vi "Measurement_input_panel.vi"(0 "OK":T4, 2 "setup":T5, 5 "Setup filename":string) -> (11 "Setup filename out":string, 12 "Analysis Info cluster":T8[](array[typedef])=[{"Colour"=0, "Inst type"=enum."Pitot-static tube", "Inst name"="Manometer voltage", "Symbol"="U", "Code name"="", "Extra Info"="U", "Inst Array"=enum."PWA", "Extra Titles"=[], "Extra Values"=[], "U"=0.0, "u^2"=0.0, "u^3"=0.0, "u^4"=0.0, "Skew_u"=0.0, "Kurt_u"=0.0, "Sd Error in Mean"=0.0, "% u'/U"=0.0, "X"=0.0, "Y"=0.0, "Z"=0.0, "Timescale integral Estimate"=0.0, "Sd Error in Variance"=0.0, "Calib File"=path "", "Calib Constants"=[], "Output Position"=FALSE, "Full Stats"=FALSE, "Av Sampling Rate"=0.0, "Av No of Samples"=0.0, "Total Meas Time (s)"=0.0, "ADAM Ch Name"="", "Max value"=0.0, "Min value"=0.0, "Req Sample Rate Hz"=0.0, "Sync Delay Time (s)"=0.0, "Ch No"=0, "Device ID"="", "Use Latest Calib"=FALSE}, {"Colour"=0, "Inst type"=enum."Pitot-static tube", "Inst name"="Manometer voltage", "Symbol"="U", "Code name"="", "Extra Info"="U", "Inst Array"=enum."PWA", "Extra Titles"=[], "Extra Values"=[], "U"=0.0, "u^2"=0.0, "u^3"=0.0, "u^4"=0.0, "Skew_u"=0.0, "Kurt_u"=0.0, "Sd Error in Mean"=0.0, "% u'/U"=0.0, "X"=0.0, "Y"=0.0, "Z"=0.0, "Timescale integral Estimate"=0.0, "Sd Error in Variance"=0.0, "Calib File"=path "", "Calib Constants"=[], "Output Position"=FALSE, "Full Stats"=FALSE, "Av Sampling Rate"=0.0, "Av No of Samples"=0.0, "Total Meas Time (s)"=0.0, "ADAM Ch Name"="", "Max value"=0.0, "Min value"=0.0, "Req Sample Rate Hz"=0.0, "Sync Delay Time (s)"=0.0, "Ch No"=0, "Device ID"="", "Use Latest Calib"=FALSE}, {"Colour"=0, "Inst type"=enum."Pitot-static tube", "Inst name"="Manometer voltage", "Symbol"="U", "Code name"="", "Extra Info"="U", "Inst Array"=enum."PWA", "Extra Titles"=[], "Extra Values"=[], "U"=0.0, "u^2"=0.0, "u^3"=0.0, "u^4"=0.0, "Skew_u"=0.0, "Kurt_u"=0.0, "Sd Error in Mean"=0.0, "% u'/U"=0.0, "X"=0.0, "Y"=0.0, "Z"=0.0, "Timescale integral Estimate"=0.0, "Sd Error in Variance"=0.0, "Calib File"=path "", "Calib Constants"=[], "Output Position"=FALSE, "Full Stats"=FALSE, "Av Sampling Rate"=0.0, "Av No of Samples"=0.0, "Total Meas Time (s)"=0.0, "ADAM Ch Name"="", "Max value"=0.0, "Min value"=0.0, "Req Sample Rate Hz"=0.0, "Sync Delay Time (s)"=0.0, "Ch No"=0, "Device ID"="", "Use Latest Calib"=FALSE}] {"Sync Delay Time (s)" format="%.4f"; "Sd Error in Variance" format="%.2f"; "Skew_u" format="%.2f"; "% u'/U" format="%.2f"; "Sd Error in Mean" format="%.2f"; "Kurt_u" format="%.2f"; "u^4" format="%.2f"; "u^3" format="%.2f"; "U" format="%.2f"; "u^2" format="%.2f"})   [LabVIEW 2017]
uses:
  Controls/Inst_type.ctl
  Controls/Analysis_info_cluster.ctl
  Controls/Instrument_Array.ctl
  Controls/LDA_Setup.ctl
  Controls/Setup.ctl
  Controls/ok_button.ctl
  Controls/Trigger_Mode.ctl
  Controls/PWA_Data.ctl
  File/Setup_Filetype.ctl
  Controls/Post_Process.ctl
  Controls/App_Global.ctl
  Globals/Meas_global.vi
  Globals/Trav_pos_global.vi
  Globals/Preference_global.vi
  Globals/Dynamic_call_global.ph.vi
panel:
  in  "Edit temp and Press":bool
  in  "Acquisition Plug in":u16(ring) items=["7HP.vi", "ADAM_Server_Channels.vi", "DataTranslation.vi", "DT_With_Multiplexer.vi", "LDA_IP.vi", "Light_Power_Reading.vi", "LJ-T7DAQ.vi", "MAGIC_Pressures.vi", "Micro-Epsilon ILD1420.vi", "Na-DAS_7609.vi", "Na-DAS_and_MAGIC_Pressures.vi", "NI-DAQmx.vi", "NI-DAQmxBaseKernel.vi", "Pressure_Multiplexer.vi", "Simulate_kernal.vi"]
  in  "Select Duplicate Channels":bool
  in  "PWA Data":T1
  out "Inst type":T2
  out "Abs Press":dbl=1013.0 format="%.1fmBar"
  out "Temp":dbl=21.0 format="%.1fC"
  in  "Trigger mode":T3
  in  "Select Plug Ins":bool
  out "XW Present?":bool
  out "Read Setup File?":bool
  out "Setup Paths":string[](array[string])
  in  "Select ADAM Channels":bool
  in  "stop":bool
  out "Notes":string
  in  "Setup filename selector":u16(ring) items=["Current_Setup.xls", "LDA_UV_157.xls", "LDA_UW_157_Mirror.xls", "Micro-Epsilon_Height.xls", "Trav_Cam_Picture.xls", "Current_Setup.xls", "LDA_UW_157_Mirror.xls", "Micro-Epsilon_Height.xls", "Trav_Cam_Picture.xls"]
  in  "Synchronise Analogue channels with LDA":bool
  in  "LDA set up":T6={"dimensions"=enum."2D", "Sampling Rate Hz"=0.1}
  in  "LDA data":enum16{"No LDA data", "Take LDA data"}(ring)=enum."Take LDA data"
  in  "Cross wire":T7(ring)
  in  "No of Analogue inst":i32=1
  in  "Ch & spans choices":T10(array[cluster]) {"Sync Delay (ms)" min=0.0; "D" format="%.2f"; "Ch No" min=0}
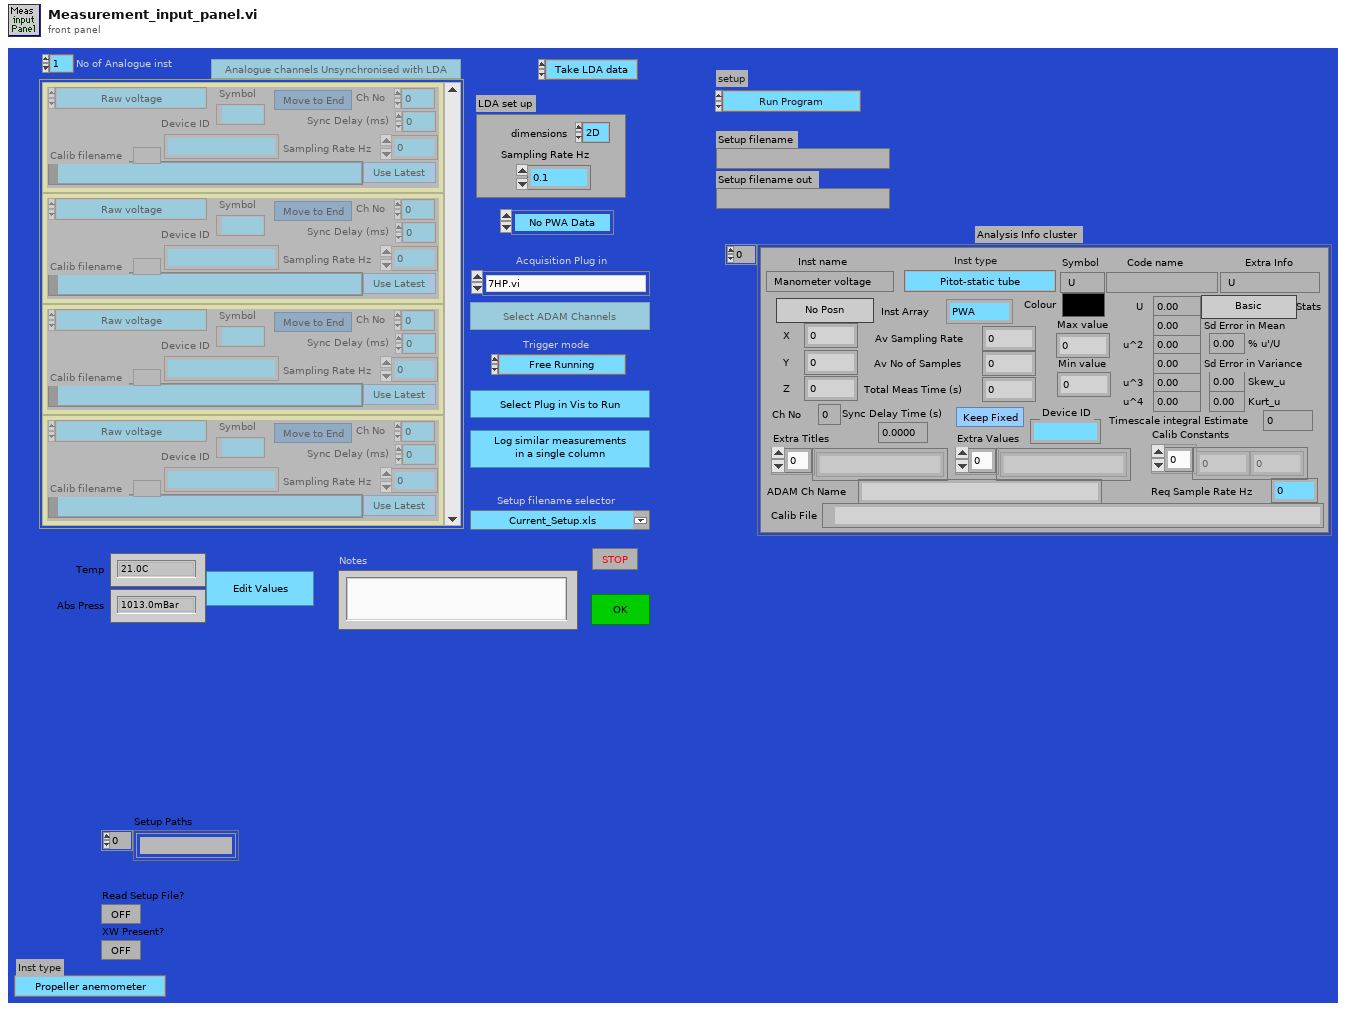
[diagram p1: front panel]
types:
  T1 = typedef "PWA_Data.ctl" = enum16{"No PWA Data", "One Ch PWA"}
  T2 = typedef "Inst_type.ctl" = enum16{"Propeller anemometer", "Raw voltage", "Pressure Transducer", "Pitot-static tube", "Preston tube", "Hot wire", "Cross wire 1", "Cross wire 2", "Generic Linear", "Generic Polynomial", "Generic BackPoly", "Fast FID", "Thermocouple", "Cold wire", "Pulsed Wire", "LDA Vel", "LDA Tran time", "LDA Arr time", "Microphone"}
  T3 = typedef "Trigger_Mode.ctl" = enum16{"Free Running", "Start on Trigger", "Trigger Every Block", "Trigger Every Sample"}
  T4 = typedef "ok_button.ctl" = bool
  T5 = typedef "Setup.ctl" = enum16{"Run Program", "Show Setup", "Save Current Setup", "Setup Front Panel"}
  T6 = typedef "LDA_Setup.ctl" = cluster{"dimensions":enum16{"1D", "2D"}, "Sampling Rate Hz":dbl}
  T7 = enum16{"2nd component as calculated", "2nd component multipled by -1"}
  T8 = typedef "Analysis_info_cluster.ctl" = cluster{"Colour":u32, "Inst type":T2, "Inst name":string, "Symbol":string, "Code name":string, "Extra Info":string, "Inst Array":T9, "Extra Titles":string[], "Extra Values":string[], "U":dbl, "u^2":dbl, "u^3":dbl, "u^4":dbl, "Skew_u":dbl, "Kurt_u":dbl, "Sd Error in Mean":dbl, "% u'/U":dbl, "X":dbl, "Y":dbl, "Z":dbl, "Timescale integral Estimate":dbl, "Sd Error in Variance":dbl, "Calib File":path, "Calib Constants":dbl[], "Output Position":bool, "Full Stats":bool, "Av Sampling Rate":dbl, "Av No of Samples":dbl, "Total Meas Time (s)":dbl, "ADAM Ch Name":string, "Max value":dbl, "Min value":dbl, "Req Sample Rate Hz":dbl, "Sync Delay Time (s)":dbl, "Ch No":i16, "Device ID":string, "Use Latest Calib":bool}
  T9 = typedef "Instrument_Array.ctl" = enum16{"PWA", "LDA", "Analogue"}
  T10 = cluster{"Ch No":i16, "Calib filename":path, "Inst type":T2, "Symbol":string, "Move channel":bool, "Use Latest":bool, "D":dbl, "Ch Name":string, "Sync Delay (ms)":dbl, "Device ID":string, "Sampling Rate Hz":dbl}[]
  T11 = typedef "Post_Process.ctl" = enum16{"Take New Data", "Post Process Raw Data File"}
  T12 = typedef "Setup_Filetype.ctl" = enum16{"Measurement Setups", "Calibration Setups", "General", "Results File Plotter Setups", "Speed Calib Tweaks"}
  T13 = typedef "App_Global.ctl" = enum16{"Read Global", "Write to Global", "Initialise Array"}
  T14 = enum16{"Zero or one", "One", "Zero or more", "One or more"}
  T15 = cluster{"Ch No":i16, "Calib filename":path, "Inst type":T2, "Symbol":string, "Move channel":bool, "Use Latest":bool, "D":dbl, "Ch Name":string, "Sync Delay (ms)":dbl, "Device ID":string, "Sampling Rate Hz":dbl}
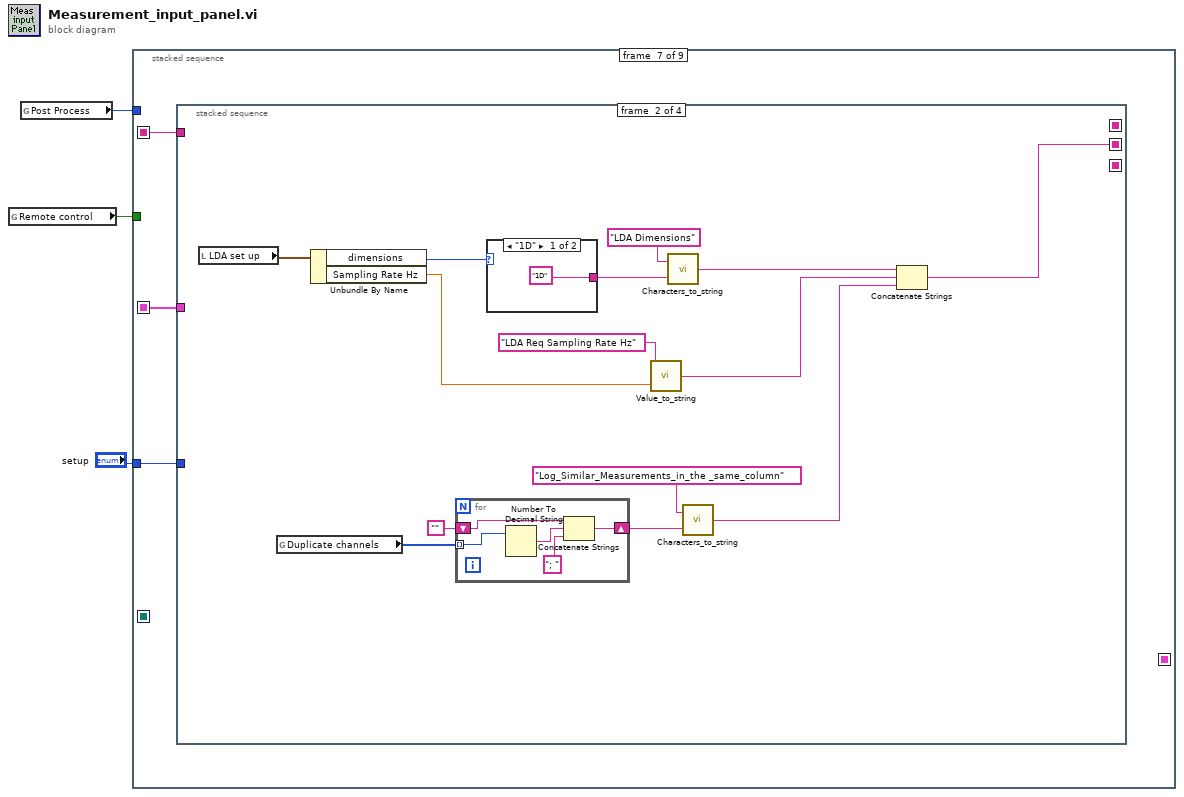
[diagram p0: block diagram]
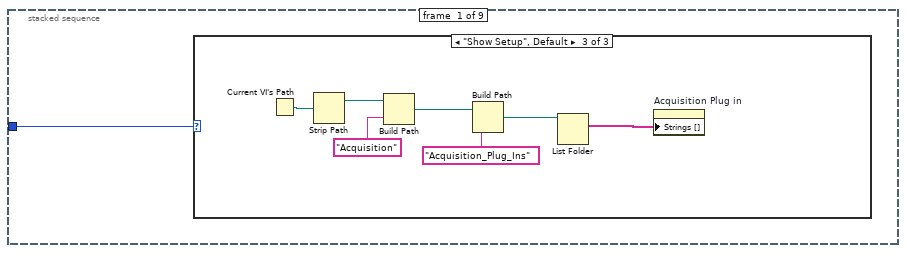
[diagram p2: hidden frame]
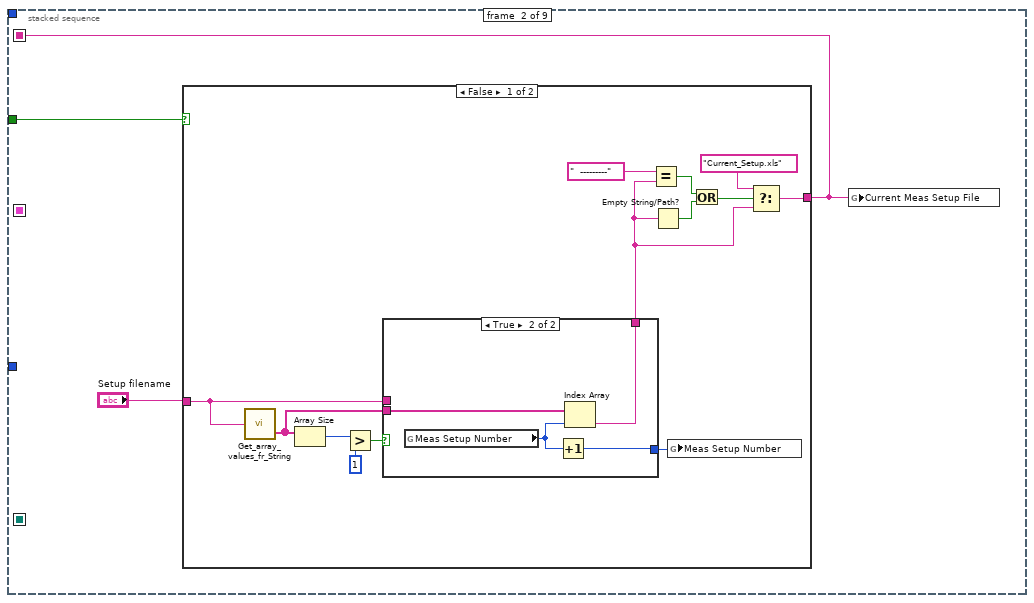
[diagram p5: hidden frame]
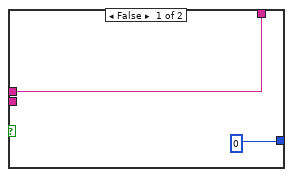
[diagram p6: hidden frame]
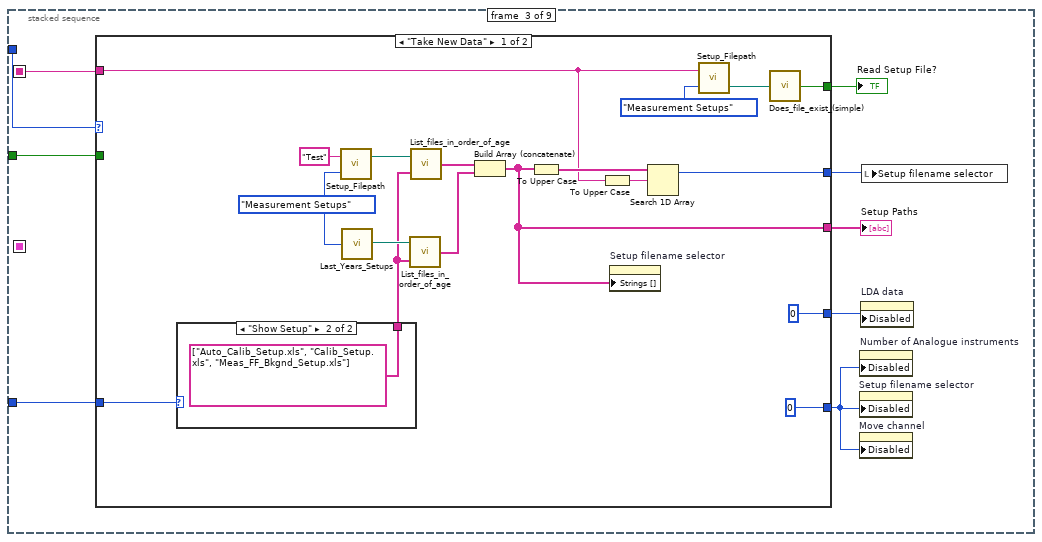
[diagram p8: hidden frame]
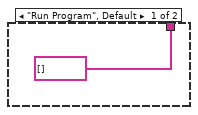
[diagram p9: hidden frame]
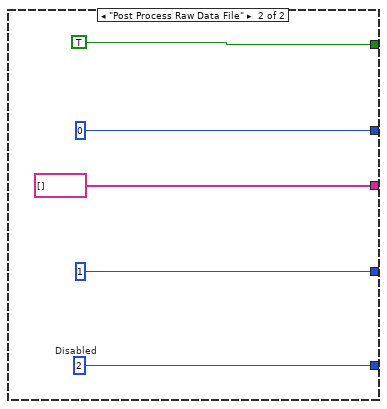
[diagram p10: hidden frame]
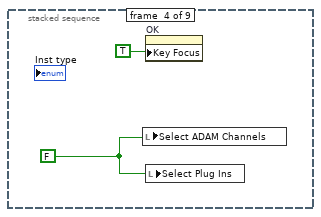
[diagram p11: hidden frame]
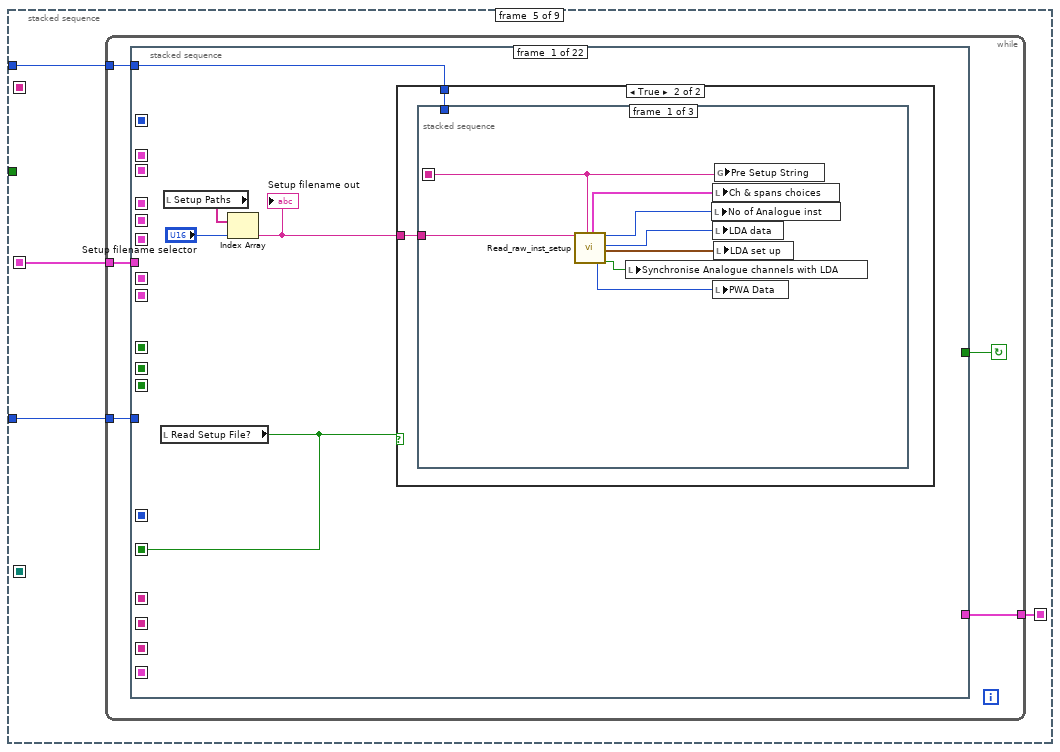
[diagram p12: hidden frame]
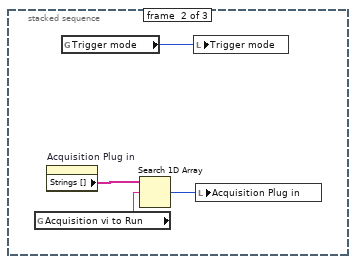
[diagram p14: hidden frame]
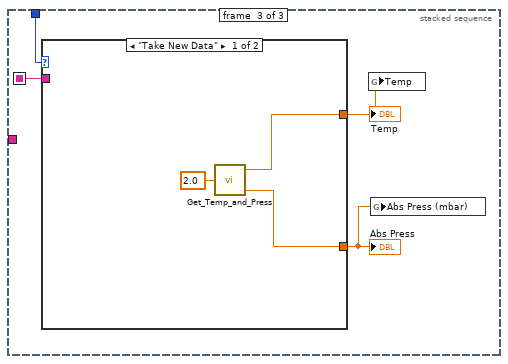
[diagram p15: hidden frame]
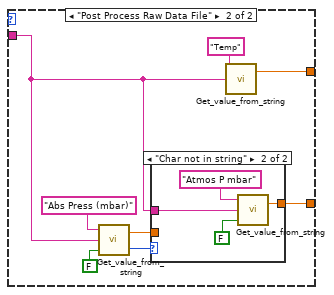
[diagram p16: hidden frame]
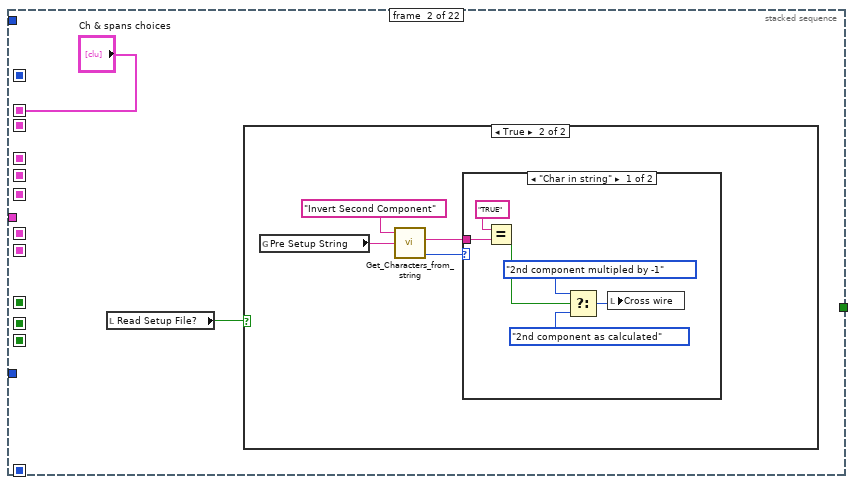
[diagram p18: hidden frame]
diagram:
  n1 = global read "Meas_global.vi" "Remote control"() -> (w1:bool)
  n2 = global read "Meas_global.vi" "Post Process"() -> (w3:T11)
  n3 = stacked-sequence {
    seq-local: [_ _ _ _ w74 _ _ _ _] -> [_ _ _ _ _ _ w699 w802 _]
    seq-local: [_ w13 _ _ _ _ _ _ _] -> [_ _ w35 _ _ _ w698 _ _]
    seq-local: [_ _ _ _ w71 _ _ _ _] -> [_ _ _ _ _ _ _ _ w855]
    seq-local: [_ _ _ _ _ _ _ w801 _] -> [_ _ _ _ _ _ _ _ w854]
    tunnel: w3 -> [_ _ w43 _ w73 _ _ w803 _]
    tunnel: "setup" -> [w4 _ w37 _ w72 _ w700 _ _]
    tunnel: w1 -> [_ w14 w36 _ _ _ _ _ _]
    frame #0 {
      n4 = case shown="\"Show Setup\", Default" w4 {
        frame "Run Program" {
        }
        frame "Setup Front Panel" {
        }
        frame "Show Setup", Default {
          n5 = Current VI's Path() -> (path=w11:path)
          n6 = Strip Path(path=w11) -> (stripped path=w10:path)  [unwired: 1 out]
          n7 = Build Path(base path=w10, name or relative path="Acquisition") -> (appended path=w7:path)
          n8 = Build Path(base path=w7, name or relative path="Acquisition_Plug_Ins") -> (appended path=w6:path)
          n9 = List Folder(path=w6) -> (filenames=w5:string[])  [unwired: 3 in, 3 out]
          n10 = property on="Acquisition Plug in" class="Ring (strict)"("Strings []"=w5) -> ()  [unwired: 2 in, 2 out]
        }
      }
    }
    frame #1 {
      n11 = case shown="False" w14 {
        tunnel: [w26 w34] -> w13
        tunnel: "Setup filename" -> [w15 w34]
        frame False {
          n12 = call "Get_array_values_fr_String.vi"("String Value"=w15) -> ("String array"=w17:string[])  [unwired: 1 out]
          n13 = Array Size(array=w17) -> (size(s)=w21:i32)
          n14 = Greater?(x=w21, y=1) -> (0:w19:bool)
          n15 = case shown="True" w19 {
            tunnel: [w29 w32] -> w18
            tunnel: w15 -> [w29 _]
            tunnel: w17 -> [_ w33]
            tunnel: [0 w30] -> w16
            frame False {
            }
            frame True {
              n16 = global read "Trav_pos_global.vi" "Meas Setup Number"() -> (w31:i32)
              n17 = Increment(x=w31) -> (x+1=w30:i32)
              n18 = Index Array(array=w33, index=w31) -> (element=w32:string)
            }
          }
          n19 = Equal?(x="  ---------" ("f"), y=w18) -> (x = y?=w25:bool)
          n20 = Empty String/Path?(string/path=w18) -> (empty?=w24:bool)
          n21 = global write "Trav_pos_global.vi" "Meas Setup Number"(w16) -> ()
          n22 = Or(x=w25, y=w24) -> (x .or. y?=w22:bool)
          n23 = Select(t="Current_Setup.xls", s=w22, f=w18) -> (s? t:f=w26:string)
        }
        frame True {
        }
      }
      n24 = global write "Trav_pos_global.vi" "Current Meas Setup File"(w13) -> ()
    }
    frame #2 {
      n25 = case shown="\"Take New Data\"" w43 {
        tunnel: [w44 string[] []] -> w39
        tunnel: [w57 TRUE ("exists")] -> w38
        tunnel: [u8 0 ("Disabled") w65] -> w40
        tunnel: [u8 0 ("Disabled") u8 1 ("Disabled")] -> w42
        tunnel: w35 -> [w53 _]
        tunnel: [w60 0 ("index of element")] -> w41
        tunnel: w37 -> [w55 _]
        tunnel: w36 -> [_ _]
        frame "Take New Data" {
          w47 = Setup_Filetype."Measurement Setups" ("Setup File Type")
          n26 = case shown="\"Show Setup\"" w55 {
            tunnel: [string[] [] ("file names") string[] ["Auto_Calib_Setup.xls", "Calib_Setup.xls", "Meas_FF_Bkgnd_Setup.xls"] ("file names")] -> w45
            frame "Run Program", Default {
            }
            frame "Show Setup" {
            }
          }
          n27 = call "Setup_Filepath.vi"("Setup File Type"=w47, "Filename in"="Test") -> ("Directory"=w48:path)  [unwired: 1 out]
          n28 = call "Last_Years_Setups.vi"("Setup File Type"=w47) -> ("Directory"=w46:path)
          n29 = call "List_files_in_order_of_age.vi"("Files to Hide"=w45, "Folder"=w46) -> ("file names"=w50:string[])
          n30 = call "List_files_in_order_of_age.vi"("Files to Hide"=w45, "Folder"=w48) -> ("file names"=w49:string[])
          n31 = Build Array (concatenate)(w49, w50) -> (w44:string[])
          n32 = To Upper Case(1:w44) -> (0:w59:string[])
          n33 = To Upper Case(1:w53) -> (0:w58:string)
          n34 = property on="Setup filename selector" class="Ring (strict)"("Strings []"=w44) -> ()  [unwired: 2 in, 2 out]
          n35 = Search 1D Array(1D array=w59, element=w58) -> (index of element=w60:i32)  [unwired: 1 out]
          n36 = call "Setup_Filepath.vi"("Setup File Type"=Setup_Filetype."Measurement Setups", "Filename in"=w53) -> ("Filename Out"=w52:path)  [unwired: 1 out]
          n37 = call "Does_file_exist_(simple).vi"("Pathname"=w52) -> ("exists?"=w57:bool)
        }
        frame "Post Process Raw Data File" {
          w65 = u8 2  # Disabled
        }
      }
      "Setup Paths" <- w39
      "Read Setup File?" <- w38
      n38 = property on="Number of Analogue instruments" class="DigNum (strict)"("Disabled"=w40) -> ()  [unwired: 2 in, 2 out]
      n39 = property on="Setup filename selector" class="Ring (strict)"("Disabled"=w40) -> ()  [unwired: 2 in, 2 out]
      n40 = property on="Move channel" class="Bool (strict)"("Disabled"=w40) -> ()  [unwired: 2 in, 2 out]
      n41 = property on="LDA data" class="Enum (strict)"("Disabled"=w42) -> ()  [unwired: 2 in, 2 out]
      n42 = local write "Setup filename selector"(w41) -> ()
    }
    frame #3 {
      w70 = FALSE ("Select Local ADAM Channels")
      n43 = local write "Select ADAM Channels"(w70) -> ()
      n44 = property on="OK" class="Bool"("Key Focus"=TRUE) -> ()  [unwired: 2 in, 2 out]
      n45 = local write "Select Plug Ins"(w70) -> ()
    }
    frame #4 {
      n46 = while {
        tunnel: w72 -> [w76]
        tunnel: w73 -> [w77]
        tunnel: [w79] -> w74
        tunnel: [w75] -> w71
        stop <- w78 continue-if-true
        n47 = stacked-sequence {
          seq-local: [_ _ _ _ _ _ _ _ w194 _ _ _ _ _ _ _ _ _ _ _ _ _] -> [_ _ _ _ _ _ _ _ _ _ w255 w280 w327 _ _ _ _ _ _ _ _ _]
          seq-local: [_ "Ch & spans choices" _ _ _ _ _ _ _ _ _ _ _ _ _ _ _ _ _ _ _ _] -> [_ _ _ _ _ w156 _ w190 w195 _ _ _ _ _ _ _ _ _ w556 _ _ _]
          seq-local: [_ _ _ _ _ w161 _ _ _ _ _ _ _ _ _ _ _ _ _ _ _ _] -> [_ _ _ _ _ _ _ _ w196 _ _ _ _ _ _ _ _ _ _ _ _ _]
          seq-local: [_ _ _ _ _ _ _ _ _ _ w257 _ _ _ _ _ _ _ _ _ _ _] -> [_ _ _ _ _ _ _ _ _ _ _ w281 _ _ _ _ _ _ _ _ _ w664]
          seq-local: [_ _ _ _ _ _ _ _ _ _ _ _ _ w359 _ _ _ _ _ _ _ _] -> [_ _ _ _ _ _ _ _ _ _ _ _ _ _ w378 _ _ _ _ _ _ _]
          seq-local: [_ _ _ _ _ _ _ _ _ _ _ _ _ _ w374 _ _ _ _ _ _ _] -> [_ _ _ _ _ _ _ _ _ _ _ _ _ _ _ w402 w472 _ _ _ w641 w665]
          seq-local: [_ _ _ _ _ _ _ _ _ _ _ w285 _ _ _ _ _ _ _ _ _ _] -> [_ _ _ _ _ _ _ _ _ _ _ _ _ w357 _ _ _ _ _ _ _ _]
          seq-local: [_ _ _ _ _ _ _ _ _ _ _ _ w331 _ _ _ _ _ _ _ _ _] -> [_ _ _ _ _ _ _ _ _ _ _ _ _ w356 _ _ _ _ _ _ _ _]
          seq-local: [_ _ _ _ _ _ _ _ _ w252 _ _ _ _ _ _ _ _ _ _ _ _] -> [_ _ _ _ _ _ _ _ _ _ w256 w282 _ _ _ _ _ _ _ _ _ w663]
          seq-local: [_ _ _ _ _ _ _ _ _ _ _ _ _ _ _ w401 _ _ _ _ _ _] -> [_ _ _ _ _ _ _ _ _ _ _ _ _ _ _ _ w475 _ _ _ _ _]
          seq-local: [_ _ _ _ _ _ _ _ _ _ _ _ _ _ _ w400 _ _ _ _ _ _] -> [_ _ _ _ _ _ _ _ _ _ _ _ _ _ _ _ w474 _ _ _ _ _]
          seq-local: [_ _ _ _ _ _ _ _ _ _ _ _ _ _ _ w399 _ _ _ _ _ _] -> [_ _ _ _ _ _ _ _ _ _ _ _ _ _ _ _ w473 _ _ _ _ _]
          seq-local: [_ _ _ _ _ _ _ _ _ _ _ _ _ _ _ _ w471 _ _ _ _ _] -> [_ _ _ _ _ _ _ _ _ _ _ _ _ _ _ _ _ _ _ w570 _ _]
          seq-local: [_ _ _ _ _ _ _ _ _ _ _ _ _ _ _ _ w469 _ _ _ _ _] -> [_ _ _ _ _ _ _ _ _ _ _ _ _ _ _ _ _ w516 _ _ _ _]
          seq-local: [w80 _ _ _ _ _ _ _ _ _ _ _ _ _ _ _ _ _ _ _ _ _] -> [_ _ _ _ _ _ _ _ _ _ _ _ _ _ _ _ w468 _ _ _ _ _]
          seq-local: [_ _ _ _ _ _ _ _ _ _ _ _ _ _ _ _ _ w515 _ _ _ _] -> [_ _ _ _ _ _ _ _ _ _ _ _ _ _ _ _ _ _ w557 _ _ _]
          seq-local: [_ _ _ _ _ _ _ _ _ _ _ _ _ _ _ _ _ _ w554 _ _ _] -> [_ _ _ _ _ _ _ _ _ _ _ _ _ _ _ _ _ _ _ w569 _ _]
          tunnel: [_ _ _ _ _ _ _ _ _ _ _ _ _ _ w374 _ _ _ _ _ _ _] -> w79
          tunnel: [_ _ _ _ _ _ _ _ _ _ _ w283 _ _ _ _ _ _ _ _ _ _] -> w78
          tunnel: w77 -> [w82 _ _ w135 _ _ _ _ _ w253 _ _ _ _ _ _ _ w526 _ _ _ _]
          tunnel: w76 -> [_ _ w131 _ w142 _ _ _ _ _ _ _ _ w358 _ _ _ _ _ w572 _ _]
          tunnel: [_ _ _ _ _ _ _ _ _ _ _ _ _ _ _ _ w471 _ _ _ _ _] -> w75
          frame #0 {
            n48 = local read "Read Setup File?"() -> (w80:bool)
            n49 = local read "Setup Paths"() -> (w84:string[])
            n50 = Index Array(array=w84, index="Setup filename selector") -> (element=w81:string)
            "Setup filename out" <- w81
            n51 = case shown="True" w80 {
              tunnel: w81 -> [_ w86]
              tunnel: w82 -> [_ w85]
              frame False {
              }
              frame True {
                n52 = stacked-sequence {
                  seq-local: [w89 _ _] -> [_ _ w101]
                  tunnel: w86 -> [w91 _ _]
                  tunnel: w85 -> [_ _ w102]
                  frame #0 {
                    n53 = call "Read_raw_inst_setup.vi"("Setup file"=w91) -> ("Setup string"=w89:string, "Ch & spans choices"=w87:T10, "PWA Data"=w88:T1, "Number of Analogue instruments"=w94:i32, "LDA data"=w93:enum16{"No LDA data", "Take LDA data"}, "LDA set up"=w90:T6, "Synchronise Analogue channels with LDA"=w92:bool)  [unwired: 12 out]
                    n54 = local write "Synchronise Analogue channels with LDA"(w92) -> ()
                    n55 = local write "No of Analogue inst"(w94) -> ()
                    n56 = local write "Ch & spans choices"(w87) -> ()
                    n57 = local write "LDA data"(w93) -> ()
                    n58 = local write "PWA Data"(w88) -> ()
                    n59 = local write "LDA set up"(w90) -> ()
                    n60 = global write "Meas_global.vi" "Pre Setup String"(w89) -> ()
                  }
                  frame #1 {
                    n61 = global read "Meas_global.vi" "Acquisition vi to Run"() -> (w96:string)
                    n62 = property on="Acquisition Plug in" class="Ring (strict)"() -> ("Strings []"=w97:string[])  [unwired: 2 in, 2 out]
                    n63 = global read "Meas_global.vi" "Trigger mode"() -> (w98:T3)
                    n64 = Search 1D Array(1D array=w97, element=w96) -> (index of element=w95:i32)  [unwired: 1 in]
                    n65 = local write "Trigger mode"(w98) -> ()
                    n66 = local write "Acquisition Plug in"(w95) -> ()
                  }
                  frame #2 {
                    n67 = case shown="\"Take New Data\"" w102 {
                      tunnel: w101 -> [_ w108]
                      tunnel: [w103 w107] -> w99
                      tunnel: [w104 w106] -> w100
                      frame "Take New Data" {
                        n68 = call "Get_Temp_and_Press.vi"("Averaging time (mins)"=2.0) -> ("Abs Press (mbar)"=w103:dbl, "Temperature"=w104:dbl)  [unwired: 3 out]
                      }
                      frame "Post Process Raw Data File" {
                        n69 = call "Get_value_from_string.vi"("Show Dialog?"=FALSE, "Input string"=w108, "Variable name"="Abs Press (mbar)") -> ("Status"=w112:enum16{"Char in string", "Char not in string"}, "Value"=w111:dbl)
                        n70 = case shown="\"Char not in string\"" w112 {
                          tunnel: [w114 w117] -> w107
                          tunnel: w111 -> [w114 _]
                          tunnel: w108 -> [_ w116]
                          frame "Char in string" {
                          }
                          frame "Char not in string" {
                            n71 = call "Get_value_from_string.vi"("Show Dialog?"=FALSE, "Input string"=w116, "Variable name"="Atmos P mbar") -> ("Value"=w117:dbl)  [unwired: 1 out]
                          }
                        }
                        n72 = call "Get_value_from_string.vi"("Input string"=w108, "Variable name"="Temp") -> ("Value"=w106:dbl)  [unwired: 1 in, 1 out]
                      }
                    }
                    "Abs Press" <- w99
                    "Temp" <- w100
                    n73 = global write "Meas_global.vi" "Temp"(w100) -> ()
                    n74 = global write "Meas_global.vi" "Abs Press (mbar)"(w99) -> ()
                  }
                }
              }
            }
          }
          frame #1 {
            n75 = local read "Read Setup File?"() -> (w120:bool)
            n76 = case shown="True" w120 {
              frame False {
              }
              frame True {
                n77 = global read "Meas_global.vi" "Pre Setup String"() -> (w123:string)
                n78 = call "Get_Characters_from_string.vi"("Input string"=w123, "Variable name"="Invert Second Component") -> ("Status"=w122:enum16{"Char in string", "Char not in string"}, "Value"=w121:string)  [unwired: 1 in]
                n79 = case shown="\"Char in string\"" w122 {
                  tunnel: w121 -> [w130 _]
                  frame "Char in string" {
                    n80 = Equal?(x="TRUE", y=w130) -> (x = y?=w126:bool)
                    n81 = Select(t=T7."2nd component multipled by -1" ("Cross wire/LDA"), s=w126, f=T7."2nd component as calculated" ("Cross wire/LDA")) -> (s? t:f=w128:T7)
                    n82 = local write "Cross wire"(w128) -> ()
                  }
                  frame "Char not in string" {
                  }
                }
              }
            }
          }
          frame #2 {
            n83 = case shown="\"Show Setup\"" w131 {
              frame "Run Program", Default {
              }
              frame "Show Setup" {
                n84 = property on="Acquisition Plug in" class="Ring (strict)"() -> ("Strings []"=w134:string[])  [unwired: 2 in, 2 out]
                n85 = Index Array(array=w134, index="Acquisition Plug in") -> (element=w132:string)
                n86 = global write "Meas_global.vi" "Acquisition vi to Run"(w132) -> ()
              }
            }
          }
          frame #3 {
            n87 = case shown="True" "Edit temp and Press" {
              tunnel: w135 -> [_ w137]
              frame False {
              }
              frame True {
                n88 = case shown="\"Take New Data\"" w137 {
                  frame "Take New Data" {
                    n89 = stacked-sequence {
                      frame #0 {
                        w138 = TRUE  # Wait until done
                        n90 = call "Run_Enter_Temp.vi"("Wait until done"=w138) -> ()  [unwired: 1 out]
                      }
                      frame #1 {
                        n91 = call "Get_Temp_and_Press.vi"("Averaging time (mins)"=2.0) -> ("Abs Press (mbar)"=w139:dbl, "Temperature"=w140:dbl)  [unwired: 3 out]
                        n92 = local write "Temp"(w140) -> ()
                        n93 = local write "Abs Press"(w139) -> ()
                      }
                    }
                  }
                  frame "Post Process Raw Data File" {
                  }
                }
              }
            }
          }
          frame #4 {
            n94 = case shown="True" "Select Plug Ins" {
              tunnel: w142 -> [_ w144]
              frame False {
              }
              frame True {
                n95 = stacked-sequence {
                  tunnel: w144 -> [w145 _]
                  frame #0 {
                    w149 = TRUE  # Show Panel?
                    n96 = global read "Meas_global.vi" "Pre Setup String"() -> (w148:string)
                    n97 = local write "Select Plug Ins"(FALSE ("Select Local ADAM Channels")) -> ()
                    n98 = call "Choose_Plug_In_to_Run.vi"("setup"=w145, "Show Panel?"=w149, "Setup String In"=w148) -> ("Setup String Out"=w147:string)  [unwired: 1 out]
                    n99 = global write "Meas_global.vi" "Pre Setup String"(w147) -> ()
                  }
                  frame #1 {
                    n100 = Current VI's Path() -> (path=w151:path)
                    n101 = call "Open_Close_Front_Panel.ph.vi"("Front Panel Window:Open"=TRUE, "VI path"=w151) -> ()  [unwired: 2 out]
                  }
                }
              }
            }
          }
          frame #5 {
            n102 = Initialize Array(0) -> (w163:i32[])  [unwired: 1 out]
            n103 = for {
              shift-right: [w170] -> w159
              shift-left: w163 -> [w171]
              tunnel: [w169] -> w157 mode=indexing
              tunnel: w156 -> [w168] mode=indexing
              tunnel: [w166] -> w155 mode=indexing
              n104 = Unbundle By Name(w168) -> ("Inst type"=w165:T2)
              n105 = case shown="\"LDA Vel\"" w165 {
                tunnel: w171 -> [w175 w179 w181 w185]
                tunnel: [w174 w178 w181 w184] -> w170
                tunnel: [FALSE TRUE FALSE FALSE] -> w169
                frame "Propeller anemometer", Default {
                  n106 = Build Array (concatenate)(w175, 1) -> (w174:i32[])
                }
                frame "Cross wire 1" {
                  n107 = Build Array (concatenate)(w179, 2) -> (w178:i32[])
                }
                frame "Cross wire 2" {
                }
                frame "LDA Vel" {
                  n108 = Build Array (concatenate)(w185, 1) -> (w184:i32[])
                }
              }
              n109 = Equal?(x=w165, y=Inst_type."Preston tube" ("Inst type")) -> (x = y?=w166:bool)
            }
            n110 = Or Array Elements(Boolean array=w155) -> (logical OR=w153:bool)
            n111 = Or Array Elements(Boolean array=w157) -> (logical OR=→"XW Present?":bool)
            n112 = property on="D" class="DigNum (strict)"("Visible"=w153) -> ()  [unwired: 2 in, 2 out]
            n113 = Build Array (concatenate)(w159, 1) -> (w158:i32[])
            n114 = Array Subset(array=w158, length="No of Analogue inst") -> (w162:i32[])  [unwired: 1 in]
            n115 = Add Array Elements(numeric array=w162) -> (sum=w161:i32)
          }
          frame #6 {
            "Notes" <- ""
          }
          frame #7 {
            n116 = Array Size(array=w190) -> (size(s)=w189:i32)
            n117 = Not Equal To 0?(x=w189) -> (x != 0?=w188:bool)
            n118 = case shown="True" w188 {
              tunnel: [enum16{"No Analogue data", "Take Analogue data"}."No Analogue data" ("Analogue data") enum16{"No Analogue data", "Take Analogue data"}."Take Analogue data" ("Analogue data")] -> w187
              frame False {
              }
              frame True {
              }
            }
            n119 = global write "Meas_global.vi" "Analogue data"(w187) -> ()
          }
          frame #8 {
            n120 = Index Array(array=w195, index=0) -> (element=w200:T15)
            n121 = Build Array (concatenate)(w195, w200) -> (w199:T10)
            n122 = Initialize Array(w200) -> (w198:T10)  [unwired: 1 out]
            n123 = for {
              N: w196 -> [_]
              tunnel: w199 -> [w208] mode=indexing
              shift-right: [w209] -> w194
              shift-left: w198 -> [w203]
              tunnel: Inst_type."Cross wire 2" ("Inst type") -> [w201]
              shift-right: [w207] -> _
              shift-left: _ -> [w206]
              tunnel: w199 -> [w205]
              n124 = Unbundle By Name(w208) -> ("Inst type"=w207:T2)
              n125 = Array Size(array=w203) -> (size(s)=w202:i32)
              n126 = Increment(x=w202) -> (x+1=w204:i32)
              n127 = case shown="\"Cross wire 1\"" w207 {
                tunnel: [w217 w237 w249] -> w209
                tunnel: w203 -> [w218 w239 w251]
                tunnel: w208 -> [w214 w240 w250]
                tunnel: w201 -> [w216 w244 _]
                tunnel: w206 -> [_ w243 _]
                tunnel: w205 -> [w221 _ _]
                tunnel: w204 -> [w220 _ _]
                frame "Cross wire 1" {
                  n128 = Index Array(array=w221, index=w220) -> (element=w215:T15)
                  n129 = Unbundle By Name(w215) -> ("Inst type"=w219:T2, "Sync Delay (ms)"=w212:dbl, "Ch No"=w211:i16, "Symbol"=w210:string)
                  n130 = Unbundle By Name(w214) -> ("Calib filename"=w213:path)
                  n131 = case shown="\"Cross wire 2\"" w219 {
                    tunnel: w218 -> [w230 w236]
                    tunnel: [w229 w235] -> w217
                    tunnel: w216 -> [w223 w231]
                    tunnel: w213 -> [w228 w234]
                    tunnel: w214 -> [w226 w232]
                    tunnel: w212 -> [w225 _]
                    tunnel: w211 -> [w224 _]
                    tunnel: w210 -> [w222 _]
                    frame "Cross wire 2" {
                      n132 = Bundle By Name(cluster=w226, "Calib filename"=w228, "Inst type"=w223, "Sync Delay (ms)"=w225, "Ch No"=w224, "Symbol"=w222) -> (w227:T15)
                      n133 = Build Array (concatenate)(w230, w226, w227) -> (w229:T10)
                    }
                    frame "Generic Linear", Default {
                      n134 = Bundle By Name(cluster=w232, "Calib filename"=w234, "Inst type"=w231) -> (w233:T15)
                      n135 = Build Array (concatenate)(w236, w232, w233) -> (w235:T10)
                    }
                  }
                }
                frame "Cross wire 2" {
                  n136 = Decrement(x=w244) -> (x-1=w242:T2)
                  n137 = Equal?(x=w242, y=w243) -> (x = y?=w241:bool)
                  n138 = Bundle By Name(cluster=w240, "Inst type"=w242) -> (w238:T15)
                  n139 = case shown="False" w241 {
                    tunnel: w239 -> [w247 w248]
                    tunnel: w238 -> [w246 _]
                    tunnel: [w245 w248] -> w237
                    frame False {
                      n140 = Build Array (concatenate)(w247, w246) -> (w245:T10)
                    }
                    frame True {
                    }
                  }
                }
                frame "Generic Linear", Default {
                  n141 = Build Array (concatenate)(w251, w250) -> (w249:T10)
                }
              }
            }
          }
          frame #9 {
            n142 = Equal?(x=w253, y=Post_Process."Take New Data" ("Post Process")) -> (x = y?=w252:bool)
          }
          frame #10 {
            n143 = case shown="True" "OK" {
              tunnel: w255 -> [_ w269]
              tunnel: [FALSE w260] -> w257
              tunnel: w256 -> [_ w261]
              frame False {
              }
              frame True {
                n144 = for {
                  tunnel: w269 -> [w279] mode=indexing
                  tunnel: [w275] -> w268 mode=indexing
                  n145 = Unbundle By Name(w279) -> ("Inst type"=w278:T2, "Symbol"=w277:string)
                  n146 = Number To Decimal String(number=w278) -> (decimal integer string=w276:string)  [unwired: 1 out]
                  n147 = Concatenate Strings(w276, w277) -> (w275:string)
                }
                n148 = call "Analyse_string_array.vi"("String array"=w268) -> ("Frequency"=w267:i32[])  [unwired: 2 out]
                n149 = Greater?(x=w267, y=1) -> (0:w265:bool[])
                n150 = global read "Meas_global.vi" "Remote control"() -> (w262:bool)
                n151 = Or Array Elements(Boolean array=w265) -> (logical OR=w264:bool)
                n152 = Compound Arithmetic op=AND(invert w262, w264, w261) -> (w263:bool)
                n153 = case shown="False" w263 {
                  tunnel: [TRUE FALSE] -> w260
                  frame False {
                  }
                  frame True {
                    n154 = Current VI's Path() -> (path=w272:path)
                    n155 = call "Open_Close_Front_Panel.ph.vi"("Front Panel Window:Open"=TRUE, "VI path"=w272) -> ()  [unwired: 2 out]
                    n156 = One Button Dialog(message="Non Unique symbol names") -> ()  [unwired: 2 out]
                  }
                }
              }
            }
          }
          frame #11 {
            n157 = And(x=w282, y=w281) -> (x .and. y?=w284:bool)
            n158 = case shown="True" w284 {
              tunnel: w280 -> [_ w293]
              tunnel: [FALSE w292] -> w285
              tunnel: [w286 w291] -> w283
              tunnel: w281 -> [w287 _]
              frame False {
                n159 = Not(x=w287) -> (.not. x?=w286:bool)
              }
              frame True {
                n160 = for {
                  shift-right: [w314] -> _
                  shift-left: string[] [] -> [w313]
                  tunnel: w293 -> [w311] mode=indexing
                  tunnel: [w302] -> w294 mode=indexing
                  shift-right: [w310] -> _
                  shift-left: path[] [] -> [w309]
                  n161 = Unbundle By Name(w311) -> ("Device ID"=w297:string, "Ch No"=w298:i16)
                  n162 = Unbundle By Name(w311) -> ("Inst type"=w308:T2, "Calib filename"=w305:path)
                  n163 = Format Into String(format string=" Ch %d", initial string=w297, w298) -> (resulting string=w295:string)  [unwired: 1 in, 1 out]
                  n164 = Equal?(x=Inst_type."Fast FID" ("Inst type"), y=w308) -> (x = y?=w301:bool)
                  n165 = Search 1D Array(1D array=w313, element=w295) -> (index of element=w312:i32)  [unwired: 1 out]
                  n166 = Search 1D Array(1D array=w309, element=w305) -> (index of element=w306:i32)  [unwired: 1 out]
                  n167 = Greater Or Equal To 0?(x=w306) -> (x >= 0?=w300:bool)
                  n168 = case shown="0, Default" w312 {
                    tunnel: w295 -> [w325 _]
                    tunnel: [w321 FALSE ("true")] -> w304
                    frame 0, Default {
                      n169 = Format Into String(format string="The Channel %s appears more than once", w325) -> (resulting string=w323:string)  [unwired: 2 in, 1 out]
                      n170 = One Button Dialog(message=w323, button name ("OK")="Ok") -> (true=w321:bool)
                    }
                    frame -1 {
                    }
                  }
                  n171 = And(x=w300, y=w301) -> (x .and. y?=w299:bool)
                  n172 = case shown="True" w299 {
                    tunnel: [w316 FALSE ("true")] -> w303
                    tunnel: w305 -> [w315 _]
                    frame True {
                      n173 = Format Into String(format string="Calibration file %s is used more than once.", w315) -> (resulting string=w318:string)  [unwired: 2 in, 1 out]
                      n174 = One Button Dialog(message=w318, button name ("OK")="Ok") -> (true=w316:bool)
                    }
                    frame False {
                    }
                  }
                  n175 = Build Array (concatenate)(w313, w295) -> (w314:string[])
                  n176 = Build Array (concatenate)(w309, w305) -> (w310:path[])
                  n177 = Or(x=w304, y=w303) -> (x .or. y?=w302:bool)
                }
                n178 = Or Array Elements(Boolean array=w294) -> (logical OR=w291:bool)
                n179 = Not(x=w291) -> (.not. x?=w292:bool)
              }
            }
          }
          frame #12 {
            n180 = call "Current_Calib_Filenames.vi"("Mode"=App_Global."Read Global") -> ("Calib Filename Out"=w328:path[], "Channel Numbers Out"=w329:i16[])  [unwired: 2 in, 1 out]
            n181 = for {
              tunnel: w327 -> [w342] mode=indexing
              tunnel: w329 -> [w344]
              tunnel: w328 -> [w343]
              tunnel: [w341] -> w331 mode=indexing
              n182 = Unbundle By Name(w342) -> ("Inst type"=w334:T2, "Ch No"=w336:i16, "Use Latest"=w337:bool, "Inst type"=w340:T2)
              n183 = Not Equal?(x=w340, y=Inst_type."Cross wire 2" ("Inst type")) -> (x != y?=w338:bool)
              n184 = Not Equal?(x=Inst_type."Raw voltage" ("Inst type"), y=w334) -> (x != y?=w332:bool)
              n185 = Compound Arithmetic op=AND(w337, w338) -> (w335:bool)
              n186 = case shown="True" w335 {
                tunnel: w344 -> [_ w355]
                tunnel: w336 -> [_ w354]
                tunnel: w343 -> [_ w352]
                tunnel: w342 -> [w345 w351]
                tunnel: [w345 w350] -> w341
                tunnel: w332 -> [_ w347]
                frame False {
                }
                frame True {
                  n187 = Search 1D Array(1D array=w355, element=w354) -> (index of element=w353:i32)  [unwired: 1 out]
                  n188 = Index Array(array=w352, index=w353) -> (element=w348:path)
                  n189 = Select(t=w348, s=w347, f=path "") -> (s? t:f=w349:path)
                  n190 = Bundle By Name(cluster=w351, "Calib filename"=w349) -> (w350:T15)
                }
              }
            }
          }
          frame #13 {
            n191 = case shown="True" w357 {
              tunnel: w356 -> [w360 w363]
              tunnel: [w360 w362] -> w359
              tunnel: w358 -> [_ w361]
              frame False {
              }
              frame True {
                n192 = case shown="\"Run Program\", Default" w361 {
                  tunnel: w363 -> [w365 w373]
                  tunnel: [w364 w373] -> w362
                  frame "Run Program", Default {
                    n193 = for {
                      tunnel: w365 -> [w366] mode=indexing
                      tunnel: [w367] -> w364 mode=indexing
                      n194 = Unbundle By Name(w366) -> ("Calib filename"=w372:path, "Use Latest"=w371:bool, "Ch No"=w370:i16, "Inst type"=w369:T2)
                      n195 = call "Find_calibration_file.vi"("Inst type"=w369, "Ch No"=w370, "Use Latest Calib"=w371, "filename"=w372) -> ("filename out"=w368:path)
                      n196 = Bundle By Name(cluster=w366, "Calib filename"=w368) -> (w367:T15)
                    }
                  }
                  frame "Setup Front Panel" {
                  }
                }
              }
            }
          }
          frame #14 {
            w376 = 0 ("Index")
            n197 = Index Array(array=w378, index=w376) -> (element=w377:T15)
            n198 = Initialize Array(w377, w376) -> (w375:T10)
            n199 = for {
              shift-right: [w386] -> w380
              shift-left: w375 -> [w385]
              shift-right: [w387] -> w381
              shift-left: w375 -> [w389]
              tunnel: w378 -> [w388] mode=indexing
              n200 = Unbundle By Name(w388) -> ("Move channel"=w390:bool)
              n201 = case shown="False" w390 {
                tunnel: w389 -> [w392 w398]
                tunnel: w388 -> [w394 w397]
                tunnel: [w393 w398] -> w387
                tunnel: [w391 w396] -> w386
                tunnel: w385 -> [w391 w395]
                frame False {
                  n202 = Build Array (concatenate)(w392, w394) -> (w393:T10)
                }
                frame True {
                  n203 = Build Array (concatenate)(w395, w397) -> (w396:T10)
                }
              }
            }
            n204 = Build Array (concatenate)(w381, w380) -> (w379:T10)
            n205 = for {
              tunnel: w379 -> [w384] mode=indexing
              tunnel: [w382] -> w374 mode=indexing
              n206 = Bundle By Name(cluster=w384, "Move channel"=FALSE) -> (w382:T15)
            }
          }
          frame #15 {
            # "#ToDo Maybe make this more generic..?"
            n207 = for {
              shift-right: [w408] -> _
              shift-left: string[] [] -> [w409]
              tunnel: [w411] -> w400 mode=indexing
              tunnel: [w405] -> w401 mode=indexing
              tunnel: w402 -> [w407] mode=indexing
              tunnel: [w404] -> w399 mode=indexing
              n208 = Unbundle By Name(w407) -> ("Inst type"=w410:T2)
              n209 = case shown="\"Raw voltage\"" w410 {
                tunnel: [w418 w422 w425 w429 w433 w437 w441 "XW" w448 w452 w457 w460 w464] -> w405
                tunnel: ["U" "P" "U" "U" "tau" "U" "U" "W" "U" "V" "C" "T" "T"] -> w412
                tunnel: w409 -> [w419 w423 w427 w431 w435 w439 w443 w445 w450 w454 w458 w462 w466]
                tunnel: [w417 w421 w426 w430 w434 w438 w442 w445 w449 w453 w456 w461 w465] -> w408
                frame "Propeller anemometer" {
                  w418 = "Prop"
                  n210 = Build Array (concatenate)(w419, w418) -> (w417:string[])
                }
                frame "Pressure Transducer" {
                  w422 = "Mano"
                  n211 = Build Array (concatenate)(w423, w422) -> (w421:string[])
                }
                frame "Raw voltage" {
                  w425 = "RV"
                  n212 = Build Array (concatenate)(w427, w425) -> (w426:string[])
                }
                frame "Pitot-static tube" {
                  w429 = "Pitot"
                  n213 = Build Array (concatenate)(w431, w429) -> (w430:string[])
                }
                frame "Preston tube" {
                  w433 = "Preston"
                  n214 = Build Array (concatenate)(w435, w433) -> (w434:string[])
                }
                frame "Hot wire" {
                  w437 = "HW"
                  n215 = Build Array (concatenate)(w439, w437) -> (w438:string[])
                }
                frame "Cross wire 1" {
                  w441 = "XW"
                  n216 = Build Array (concatenate)(w443, w441) -> (w442:string[])
                }
                frame "Cross wire 2" {
                }
                frame "Generic Linear", Default {
                  w448 = "Gen"
                  n217 = Build Array (concatenate)(w450, w448) -> (w449:string[])
                }
                frame "Microphone" {
                  w452 = "Mic"
                  n218 = Build Array (concatenate)(w454, w452) -> (w453:string[])
                }
                frame "Fast FID" {
                  w457 = "FF"
                  n219 = Build Array (concatenate)(w458, w457) -> (w456:string[])
                }
                frame "Thermocouple" {
                  w460 = "T"
                  n220 = Build Array (concatenate)(w462, w460) -> (w461:string[])
                }
                frame "Cold wire" {
                  w464 = "CW"
                  n221 = Build Array (concatenate)(w466, w464) -> (w465:string[])
                }
              }
              n222 = call "Analyse_string_array.vi"("String array"=w408) -> ("Unique strings"=w416:string[], "Frequency"=w414:i32[])  [unwired: 1 out]
              n223 = Search 1D Array(1D array=w416, element=w405) -> (index of element=w415:i32)  [unwired: 1 out]
              n224 = Index Array(array=w414, index=w415) -> (element=w406:i32)
              n225 = Number To Decimal String(number=w406) -> (decimal integer string=w404:string)  [unwired: 1 out]
              n226 = Concatenate Strings(w404, w405, ":", w412) -> (w411:string)
            }
          }
          frame #16 {
            w476 = T8 {"Colour"=0, "Inst type"=enum."Pitot-static tube", "Inst name"="Manometer voltage", "Symbol"="U", "Code name"="", "Extra Info"="U", "Inst Array"=enum."PWA", "Extra Titles"=[], "Extra Values"=[], "U"=0.0, "u^2"=0.0, "u^3"=0.0, "u^4"=0.0, "Skew_u"=0.0, "Kurt_u"=0.0, "Sd Error in Mean"=0.0, "% u'/U"=0.0, "X"=0.0, "Y"=0.0, "Z"=0.0, "Timescale integral Estimate"=0.0, "Sd Error in Variance"=0.0, "Calib File"=path "", "Calib Constants"=[], "Output Position"=FALSE, "Full Stats"=FALSE, "Av Sampling Rate"=0.0, "Av No of Samples"=0.0, "Total Meas Time (s)"=0.0, "ADAM Ch Name"="", "Max value"=0.0, "Min value"=0.0, "Req Sample Rate Hz"=0.0, "Sync Delay Time (s)"=0.0, "Ch No"=0, "Device ID"="", "Use Latest Calib"=FALSE}  # Analysis info cluster
            n227 = global read "Meas_global.vi" "Pre Setup String"() -> (w470:string)
            n228 = for {
              tunnel: w472 -> [w490] mode=indexing
              tunnel: w475 -> [w504] mode=indexing
              tunnel: [w506] -> w471 mode=indexing
              tunnel: w474 -> [w493] mode=indexing
              tunnel: w476 -> [w505]
              tunnel: w473 -> [w501] mode=indexing
              tunnel: w470 -> [w494]
              tunnel: [w489] -> w469 mode=indexing
              tunnel: w468 -> [w485]
              n229 = Unbundle By Name(w490) -> ("Use Latest"=w477:bool, "Sync Delay (ms)"=w483:dbl, "Ch No"=w478:i16, "Inst type"=w499:T2, "Symbol"=w498:string, "D"=w497:dbl, "Ch Name"=w486:string, "Device ID"=w480:string, "Sampling Rate Hz"=w479:dbl)
              n230 = Empty String/Path?(string/path=w498) -> (empty?=w502:bool)
              n231 = Concatenate Strings(w493, "_ADAM_Ch_Name" ("string")) -> (w491:string)
              n232 = Select(t=w501, s=w502, f=w498) -> (s? t:f=w500:string)
              n233 = Format Into String(format string="%s (%s)" ("Format String"), w504, w500) -> (resulting string=w495:string)  [unwired: 2 in, 1 out]
              n234 = call "Get_Characters_from_string.vi"("Input string"=w494, "Variable name"=w491) -> ("Value"=w488:string)  [unwired: 1 in, 1 out]
              n235 = Select(t=w488, s=w485, f=w486) -> (s? t:f=w487:string)
              n236 = Bundle By Name(cluster=w490, "Ch Name"=w487) -> (w489:T15)
              n237 = case shown="\"Preston tube\"" w499 {
                tunnel: [w509 w512] -> w481
                tunnel: w478 -> [w507 _]
                tunnel: w497 -> [_ w510]
                frame "Propeller anemometer", Default {
                  n238 = Format Into String(format string="Ch %d" ("Format String"), w507) -> (resulting string=w509:string)  [unwired: 2 in, 1 out]
                }
                frame "Preston tube" {
                  n239 = Format Into String(format string="D = %.2f" ("Format String"), w510) -> (resulting string=w512:string)  [unwired: 2 in, 1 out]
                }
              }
              n240 = Divide(x=w483, y=1000.0) -> (x/y=w482:dbl)
              n241 = Bundle By Name(cluster=w505, "Use Latest Calib"=w477, "Extra Info"=w481, "Device ID"=w480, "Inst type"=w499, "Inst name"=w495, "Symbol"=w500, "Code name"=w493, "Inst Array"=Instrument_Array."Analogue", "ADAM Ch Name"=w487, "Sync Delay Time (s)"=w482, "Req Sample Rate Hz"=w479, "Ch No"=w478) -> (w506:T8)
            }
          }
          frame #17 {
            w523 = u8 0  # Disabled
            n242 = global read "Meas_global.vi" "Acquisition vi to Run"() -> (w519:string)
            n243 = local read "Read Setup File?"() -> (w520:bool)
            n244 = Equal?(x="ADAM_Server_Channels.vi", y=w519) -> (x = y?=w517:bool)
            n245 = And(x=w520, y=w517) -> (x .and. y?=w529:bool)
            n246 = Or(x="Select ADAM Channels", y=w529) -> (x .or. y?=w524:bool)
            n247 = Equal?(x=w526, y=Post_Process."Take New Data" ("Post Process")) -> (x = y?=w525:bool)
            n248 = And(x=w525, y=w524) -> (x .and. y?=w514:bool)
            n249 = case shown="True" w514 {
              tunnel: [w530 w531] -> w515
              tunnel: w516 -> [w530 w534]
              tunnel: "Select ADAM Channels" -> [_ w533]
              tunnel: w517 -> [_ w532]
              frame False {
              }
              frame True {
                n250 = stacked-sequence {
                  seq-local: [w536 _ _] -> [_ w546 _]
                  tunnel: w534 -> [w538 w545 _]
                  tunnel: [_ w543 _] -> w531
                  tunnel: w533 -> [w540 _ w552]
                  tunnel: w532 -> [w539 _ _]
                  frame #0 {
                    n251 = Not(x=w539) -> (.not. x?=w535:bool)
                    n252 = Array Size(array=w538) -> ()  [unwired: 1 out]
                    n253 = for {
                      tunnel: w538 -> [w542] mode=indexing
                      tunnel: [w541] -> w537 mode=indexing
                      n254 = Unbundle By Name(w542) -> ("Ch Name"=w541:string)
                    }
                    n255 = call "Get_local_ADAM_Chs.vi"("Local ADAM?"=w535, "Show setup"=w540, "Desired ADAM Channels"=w537) -> ("Chosen Channels"=w536:string[])  [unwired: 1 out]
                  }
                  frame #1 {
                    n256 = for {
                      tunnel: [w551] -> w543 mode=indexing
                      tunnel: w546 -> [w550] mode=indexing
                      tunnel: w545 -> [w549]
                      i -> [w548]
                      n257 = Index Array(array=w549, index=w548) -> (element=w547:T15)
                      n258 = Bundle By Name(cluster=w547, "Ch No"=w548, "Ch Name"=w550) -> (w551:T15)
                    }
                    n259 = Array Size(array=w543) -> (size(s)=w544:i32)
                    n260 = local write "No of Analogue inst"(w544) -> ()
                  }
                  frame #2 {
                    n261 = case shown="True" w552 {
                      frame False {
                      }
                      frame True {
                        n262 = local write "Select ADAM Channels"(FALSE ("Select Local ADAM Channels")) -> ()
                      }
                    }
                  }
                }
              }
            }
            n263 = Not(x=w517) -> (.not. x?=w513:bool)
            n264 = Select(t=w523, s=w517, f=u8 2 ("Disabled")) -> (s? t:f=w521:u8)
            n265 = property on="Select ADAM Channels" class="Bool (strict)"("Disabled"=w521) -> ()  [unwired: 2 in, 2 out]
            n266 = property on="Ch Name" class="Str"("Visible"=w517) -> ()  [unwired: 2 in, 2 out]
            n267 = property on="Ch No" class="DigNum (strict)"("Visible"=w513) -> ()  [unwired: 2 in, 2 out]
            n268 = property on="Device ID" class="Str"("Visible"=w513) -> ()  [unwired: 2 in, 2 out]
            n269 = property on="Sampling Rate Hz" class="DigNum (strict)"("Visible"=w513) -> ()  [unwired: 2 in, 2 out]
          }
          frame #18 {
            n270 = Not Equal?(x=w556, y=w557) -> (x != y?=w558:bool)
            n271 = local read "LDA data"() -> (w555:enum16{"No LDA data", "Take LDA data"})
            n272 = case shown="True" w558 {
              tunnel: w557 -> [_ w565]
              frame False {
              }
              frame True {
                n273 = local write "Ch & spans choices"(w565) -> ()
              }
            }
            n274 = case shown="\"Take LDA data\"" w555 {
              tunnel: [0 w560] -> w554
              frame "No LDA data" {
              }
              frame "Take LDA data" {
                n275 = local read "LDA set up"() -> (w562:T6)
                n276 = Unbundle By Name(w562) -> ("dimensions"=w561:enum16{"1D", "2D"})
                n277 = case shown="\"2D\"" w561 {
                  tunnel: [1 2] -> w560
                  frame "1D" {
                  }
                  frame "2D" {
                  }
                }
              }
            }
          }
          frame #19 {
            n278 = global read "Meas_global.vi" "Duplicate channels"() -> (w568:i32[])
            n279 = case shown="False" "Select Duplicate Channels" {
              tunnel: w572 -> [_ _]
              tunnel: w570 -> [w583 w607]
              tunnel: w568 -> [w577 w609]
              tunnel: [w576 w608] -> w567
              tunnel: w569 -> [w575 w606]
              frame False {
                n280 = for {
                  tunnel: w583 -> [w603] mode=indexing
                  tunnel: [w602] -> w574 mode=indexing
                  n281 = Unbundle By Name(w603) -> ("Inst type"=w602:T2)
                }
                n282 = case shown="1" w575 {
                  tunnel: [w592 w594 w597] -> w573
                  tunnel: w574 -> [w592 w595 w598]
                  frame 0, Default {
                  }
                  frame 1 {
                    n283 = Build Array (concatenate)(Inst_type."LDA Vel" ("Inst type"), w595) -> (w594:T2[])
                  }
                  frame 2 {
                    w596 = Inst_type."LDA Vel" ("Inst type")
                    n284 = Build Array (concatenate)(w596, w596, w598) -> (w597:T2[])
                  }
                }
                n285 = for {
                  tunnel: w577 -> [w599] mode=indexing
                  tunnel: w573 -> [w601]
                  tunnel: [w600] -> w587 mode=indexing
                  tunnel: [w599] -> w584 mode=indexing
                  n286 = Index Array(array=w601, index=w599) -> (element=w600:T2)
                }
                n287 = Array Size(array=w573) -> (size(s)=w585:i32)
                n288 = Array Max & Min(array=w587) -> (max value=w588:T2, min value=w589:T2)  [unwired: 2 out]
                n289 = Array Max & Min(array=w584) -> (max index (indices)=w586:i32)  [unwired: 3 out]
                n290 = Array Size(array=w577) -> (size(s)=w582:i32)
                n291 = Greater?(x=w582, y=1) -> (0:w579:bool)
                n292 = Equal?(x=w588, y=w589) -> (x = y?=w591:bool)
                n293 = Greater?(x=w585, y=w586) -> (0:w590:bool)
                n294 = Compound Arithmetic op=AND(w579, w591, w590) -> (w578:bool)
                n295 = Select(t=w577, s=w578, f=i32[] [] ("32bit integer")) -> (s? t:f=w576:i32[])
              }
              frame True {
                n296 = for {
                  tunnel: w607 -> [w625] mode=indexing
                  tunnel: [w624] -> w604 mode=indexing
                  n297 = Unbundle By Name(w625) -> ("Inst name"=w624:string)
                }
                n298 = case shown="1" w606 {
                  tunnel: [w616 w618 w622] -> w605
                  tunnel: w604 -> [w616 w619 w623]
                  frame 0, Default {
                  }
                  frame 1 {
                    n299 = Build Array (concatenate)("1st LDA Ch", w619) -> (w618:string[])
                  }
                  frame 2 {
                    n300 = Build Array (concatenate)("1st LDA Ch", "2nd LDA Ch", w623) -> (w622:string[])
                  }
                }
                n301 = for {
                  shift-right: [w627] -> w612
                  shift-left: string[] [] -> [w628]
                  tunnel: w609 -> [w630]
                  tunnel: [w626] -> w611 mode=indexing
                  tunnel: w605 -> [w626] mode=indexing
                  i -> [w631]
                  n302 = Search 1D Array(1D array=w630, element=w631) -> (index of element=w629:i32)  [unwired: 1 out]
                  n303 = case shown="0, Default" w629 {
                    tunnel: w628 -> [w634 w635]
                    tunnel: w626 -> [w633 _]
                    tunnel: [w632 w635] -> w627
                    frame 0, Default {
                      n304 = Build Array (concatenate)(w634, w633) -> (w632:string[])
                    }
                    frame -1 {
                    }
                  }
                }
                n305 = local write "Select Duplicate Channels"(FALSE ("Select Local ADAM Channels")) -> ()
                n306 = call "Select_Strings.vi"("Available Ch names"=w611, "Message"="Please select similar instruments whose results columns will be combined", "Selector mode"=T14."Zero or more", "Desired Ch names (in)"=w612) -> ("Ch Indicies Chosen"=w608:i32[])  [unwired: 1 in, 3 out]
              }
            }
            n307 = global write "Meas_global.vi" "Duplicate ch being Analysed"(-1 ("Duplicate ch being Analysed")) -> ()
            n308 = global write "Meas_global.vi" "Duplicate channels"(w567) -> ()
          }
          frame #20 {
            n309 = case shown="\"Take LDA data\"" "LDA data" {
              tunnel: [w646 w649] -> w640
              tunnel: w641 -> [_ w647]
              tunnel: [w646 w648] -> w637
              frame "No LDA data" {
                w646 = u8 2  # Disabled
                n310 = local write "Synchronise Analogue channels with LDA"(FALSE ("Synchronise Analogue channels with LDA")) -> ()
              }
              frame "Take LDA data" {
                n311 = stacked-sequence {
                  tunnel: [w650 _] -> w649
                  tunnel: [_ w652] -> w648
                  tunnel: w647 -> [_ w653]
                  frame #0 {
                    w650 = u8 0  # Disabled
                  }
                  frame #1 {
                    n312 = Array Size(array=w653) -> (size(s)=w654:i32)
                    n313 = Not Equal To 0?(x=w654) -> (x != 0?=w651:bool)
                    n314 = case shown="False" w651 {
                      selector: w651 -> [w655 _]
                      tunnel: [u8 2 ("Disabled") u8 0 ("Disabled")] -> w652
                      frame False {
                        n315 = local write "Synchronise Analogue channels with LDA"(w655) -> ()
                      }
                      frame True {
                      }
                    }
                  }
                }
              }
            }
            n316 = local read "XW Present?"() -> (w638:bool)
            n317 = case shown="False" w638 {
              tunnel: [w643 "Cross wire"] -> w636
              frame False {
                w643 = T7."2nd component as calculated"  # Cross wire/LDA
              }
              frame True {
              }
            }
            n318 = property on="Cross wire/LDA" class="Enum (strict)"("Visible"=w638) -> ()  [unwired: 2 in, 2 out]
            n319 = global write "Meas_global.vi" "Cross wire + or -ve"(w636) -> ()
            n320 = property on="LDA set up" class="Clust (strict)"("Disabled"=w640) -> ()  [unwired: 2 in, 2 out]
            n321 = property on="Synchronise Analogue channels with LDA" class="Bool (strict)"("Disabled"=w637) -> ()  [unwired: 2 in, 2 out]
            n322 = Wait (ms)(milliseconds to wait=u32 100) -> ()  [unwired: 1 out]
          }
          frame #21 {
            n323 = And(x=w663, y=w664) -> (x .and. y?=w662:bool)
            n324 = local read "Synchronise Analogue channels with LDA"() -> (w661:bool)
            n325 = while {
              shift-left: _ -> [w690]
              shift-right: [w691] -> w658
              tunnel: [w692] -> w660
              stop <- FALSE continue-if-true
              n326 = local read "Setup filename selector"() -> (w691:u16)
              n327 = Not Equal?(x=w691, y=w690) -> (x != y?=w692:bool)
            }
            n328 = case shown="True" w661 {
              tunnel: w665 -> [_ w676]
              tunnel: w662 -> [_ w675]
              frame False {
              }
              frame True {
                n329 = case shown="True" w675 {
                  tunnel: w676 -> [_ w679]
                  frame False {
                  }
                  frame True {
                    n330 = for {
                      tunnel: w679 -> [w688] mode=indexing
                      tunnel: [w681] -> w678 mode=indexing
                      n331 = Unbundle By Name(w688) -> ("Inst type"=w687:T2, "Symbol"=w685:string)
                      n332 = Equal?(x=w685, y="Sync") -> (x = y?=w683:bool)
                      n333 = Equal?(x=Inst_type."Raw voltage" ("Inst type"), y=w687) -> (x = y?=w682:bool)
                      n334 = And(x=w682, y=w683) -> (x .and. y?=w681:bool)
                    }
                    n335 = Or Array Elements(Boolean array=w678) -> (logical OR=w677:bool)
                    n336 = case shown="False" w677 {
                      frame False {
                        n337 = One Button Dialog(message="To Perform LDA Sync you must provide a Raw voltage channel having the symbol \"Sync\"") -> ()  [unwired: 2 out]
                      }
                      frame True {
                      }
                    }
                  }
                }
              }
            }
            n338 = case shown="True" w660 {
              tunnel: [FALSE ("exists?") w674] -> w659
              tunnel: w658 -> [_ w672]
              frame False {
              }
              frame True {
                n339 = local read "Setup Paths"() -> (w673:string[])
                n340 = Index Array(array=w673, index=w672) -> (element=w670:string)
                n341 = call "Setup_Filepath.vi"("Setup File Type"=Setup_Filetype."Measurement Setups", "Filename in"=w670) -> ("Filename Out"=w669:path)  [unwired: 1 out]
                n342 = call "Does_file_exist_(simple).vi"("Pathname"=w669) -> ("exists?"=w674:bool)
              }
            }
            n343 = local write "Read Setup File?"(w659) -> ()
            n344 = Current VI's Path() -> (path=w666:path)
            n345 = call "Close_Panel_and_Abort.vi"("Vi path"=w666, "stop"="stop") -> ()  [unwired: 1 out]
          }
        }
      }
    }
    frame #5 {
      n346 = local read "LDA data"() -> (w695:enum16{"No LDA data", "Take LDA data"})
      n347 = case shown="\"Take LDA data\"" w695 {
        tunnel: [FALSE ("Synchronise Analogue channels with LDA") "Synchronise Analogue channels with LDA"] -> w694
        frame "No LDA data" {
        }
        frame "Take LDA data" {
        }
      }
      n348 = global write "Meas_global.vi" "LDA data"(w695) -> ()
      n349 = global write "Meas_global.vi" "LDA set up"("LDA set up") -> ()
      n350 = global write "Meas_global.vi" "Synchronise with LDA"(w694) -> ()
    }
    frame #6 {
      n351 = stacked-sequence {
        seq-local: [_ w735 _ _] -> [_ _ _ w795]
        seq-local: [_ _ w761 _] -> [_ _ _ w794]
        seq-local: [w703 _ _ _] -> [_ _ _ w786]
        tunnel: w700 -> [w702 _ _ w789]
        tunnel: w699 -> [_ _ _ w788]
        tunnel: w698 -> [w701 _ _ _]
        frame #0 {
          n352 = local read "PWA Data"() -> (w704:T1)
          n353 = case shown="\"One Ch PWA\"" w704 {
            tunnel: ["" w713] -> w703
            tunnel: w702 -> [_ w712]
            tunnel: w701 -> [_ w708]
            frame "No PWA Data" {
            }
            frame "One Ch PWA" {
              n354 = Not Equal?(x="Calib_Setup.xls", y=w708) -> (x != y?=w707:bool)
              n355 = case shown="\"Setup Front Panel\"" w712 {
                tunnel: [w717 w720 w723 w726] -> w711
                tunnel: [w716 w719 w722 w725] -> w710
                tunnel: [w715 w718 w721 w724] -> w706
                tunnel: w707 -> [w715 w718 w721 _]
                frame "Show Setup" {
                  w717 = TRUE  # Show Panel?
                  w716 = T4 FALSE  # OK
                }
                frame "Run Program" {
                  w720 = FALSE  # Show Panel?
                  w719 = T4 TRUE  # OK
                }
                frame "Save Current Setup" {
                  w723 = FALSE  # Show Panel?
                  w722 = T4 TRUE  # OK
                }
                frame "Setup Front Panel" {
                  w724 = FALSE  # Check Calib file?
                  w726 = FALSE  # Show Panel?
                  w725 = T4 TRUE  # OK
                }
              }
              n356 = global read "Meas_global.vi" "Pre Setup String"() -> (w714:string)
              n357 = call "PWA_Setup_Panel.vi"("Show Panel?"=w711, "Check Calib file?"=w706, "OK"=w710, "Incoming Setup String"=w714) -> ("Outgoing Setup String"=w713:string)  [unwired: 3 out]
            }
          }
        }
        frame #1 {
          n358 = local read "LDA set up"() -> (w740:T6)
          n359 = global read "Meas_global.vi" "Duplicate channels"() -> (w739:i32[])
          n360 = Unbundle By Name(w740) -> ("dimensions"=w732:enum16{"1D", "2D"}, "Sampling Rate Hz"=w730:dbl)
          n361 = for {
            shift-right: [w743] -> w737
            shift-left: "" -> [w746]
            tunnel: w739 -> [w747] mode=indexing
            n362 = Number To Decimal String(number=w747) -> (decimal integer string=w745:string)  [unwired: 1 out]
            n363 = Concatenate Strings(w746, w745, "; ") -> (w743:string)
          }
          n364 = case shown="\"1D\"" w732 {
            tunnel: ["1D" "2D"] -> w734
            frame "1D" {
            }
            frame "2D" {
            }
          }
          n365 = call "Value_to_string.vi"("Value"=w730, "Label for value"="LDA Req Sampling Rate Hz") -> ("Output string"=w728:string)  [unwired: 1 in]
          n366 = call "Characters_to_string.vi"("Characters to write"=w734, "Label for characters"="LDA Dimensions") -> ("Output string"=w733:string)
          n367 = call "Characters_to_string.vi"("Characters to write"=w737, "Label for characters"="Log_Similar_Measurements_in_the _same_column") -> ("Output string"=w729:string)
          n368 = Concatenate Strings(w733, w728, w729) -> (w735:string)
        }
        frame #2 {
          n369 = global read "Preference_global.vi" "Rig Setup"() -> (w750:string)
          n370 = local read "Cross wire"() -> (w764:T7)
          n371 = case shown="\"Trigger Every Sample\"" "Trigger mode" {
            tunnel: ["Free Running" "Trigger Every Block" "Trigger Every Sample" "Start on Trigger"] -> w759
            frame "Free Running" {
            }
            frame "Trigger Every Block" {
            }
            frame "Trigger Every Sample" {
            }
            frame "Start on Trigger" {
            }
          }
          n372 = global write "Meas_global.vi" "Trigger mode"("Trigger mode") -> ()
          n373 = Match Pattern(string=w750, regular expression="-") -> (before substring=w749:string)  [unwired: 4 out]
          n374 = property on="PWA Data" class="Enum (strict)"() -> ("Strings []"=w755:string[])  [unwired: 2 in, 2 out]
          n375 = Equal?(x=T7."2nd component multipled by -1" ("Cross wire/LDA"), y=w764) -> (x = y?=w763:bool)
          n376 = case shown="\"EnFlo_Tunnel\"" w749 {
            tunnel: ["" w771] -> w748
            frame "False", Default {
            }
            frame "EnFlo_Tunnel" {
              n377 = call "Characters_to_string.vi"("Characters to write"="FALSE", "Label for characters"="Show_all_EnFlo_Tunnel_Columns") -> ("Output string"=w771:string)
            }
          }
          n378 = global write "Meas_global.vi" "PWA Data"("PWA Data") -> ()
          n379 = Index Array(array=w755, index="PWA Data") -> (element=w754:string)
          n380 = Select(t="TRUE", s=w763, f="FALSE") -> (s? t:f=w766:string)
          n381 = call "Characters_to_string.vi"("Characters to write"=w754, "Label for characters"="Pulsed_Wire_Data" ("Variable name")) -> ("Output string"=w753:string)
          n382 = call "Characters_to_string.vi"("Characters to write"=w766, "Label for characters"="Invert Second Component") -> ("Output string"=w762:string)
          n383 = call "Characters_to_string.vi"("Characters to write"=w759, "Label for characters"="Trigger mode") -> ("Output string"=w757:string)
          n384 = Concatenate Strings(w757, w753, w762, w748) -> (w761:string)
        }
        frame #3 {
          w778 = "Pre_Analysis_Plugin" ("Variable name")
          w790 = FALSE  # Show Panel?
          n385 = global read "Meas_global.vi" "Pre Setup String"() -> (w783:string)
          n386 = for {
            tunnel: w788 -> [w800] mode=indexing
            tunnel: [w799] -> w785 mode=indexing
            n387 = Unbundle By Name(w800) -> ("Ch Name"=w799:string)
          }
          n388 = call "Get_Characters_from_string.vi"("Show Dialog?"=FALSE, "Input string"=w783, "Variable name"=w778) -> ("Value"=w782:string)  [unwired: 1 out]
          n389 = global write "Dynamic_call_global.ph.vi" "Pre_Analysis_Plugin"(w782) -> ()
          n390 = Array To Spreadsheet String(array=w785, 3:"%s" ("format string")) -> (spreadsheet string=w787:string)  [unwired: 1 out]
          n391 = call "Choose_Plug_In_to_Run.vi"("setup"=w789, "Show Panel?"=w790, "Setup String In"=w783) -> ("Setup String Out"=w791:string)  [unwired: 1 out]
          n392 = call "Date_and_Time_to_string.vi"() -> ("Date and time (spreadsheet)"=w793:string)
          n393 = call "Add_label_to_string.vi"("String to write"=w787, "File Label"="Local ADAM Channels") -> ("Output string"=w796:string)
          n394 = call "Characters_to_string.vi"("Characters to write"="", "Label for characters"=w778) -> ("Output string"=w779:string)
          n395 = global read "Meas_global.vi" "New Setup String"() -> (w792:string)
          n396 = Concatenate Strings(w792, w786, w791, w793, w795, w794, w796, w779) -> (w798:string)
          n397 = global write "Meas_global.vi" "New Setup String"(w798) -> ()
        }
      }
    }
    frame #7 {
      n398 = case shown="\"Take New Data\"" w803 {
        tunnel: w802 -> [w810 w846]
        tunnel: [w804 w840] -> w801
        frame "Take New Data" {
          n399 = for {
            tunnel: w810 -> [w822] mode=indexing
            shift-right: [w818] -> w807
            shift-left: i16[] [] -> [w820]
            shift-right: [w816] -> w806
            shift-left: path[] [] -> [w817]
            tunnel: [w813] -> w804 mode=indexing
            n400 = Unbundle By Name(w822) -> ("Use Latest"=w815:bool, "Inst type"=w821:T2, "Ch No"=w819:i16, "Calib filename"=w814:path)
            n401 = call "Current_Filepath.vi"("Short_Name"="Cal" ("Data Type"), "Filename in"=w814, "Data Type"="Calibrations") -> ("Filename Out"=w813:path)  [unwired: 1 in, 1 out]
            n402 = case shown="\"Propeller anemometer\", Default" w821 {
              tunnel: w820 -> [w829 w839]
              tunnel: w819 -> [w828 _]
              tunnel: [w827 w839] -> w818
              tunnel: w817 -> [w826 w838]
              tunnel: w814 -> [w825 _]
              tunnel: [w824 w838] -> w816
              tunnel: w815 -> [w823 _]
              frame "Propeller anemometer", Default {
                n403 = case shown="False" w823 {
                  tunnel: w829 -> [w835 w837]
                  tunnel: w828 -> [w834 _]
                  tunnel: [w833 w837] -> w827
                  tunnel: w826 -> [w832 w836]
                  tunnel: w825 -> [w831 _]
                  tunnel: [w830 w836] -> w824
                  frame False {
                    n404 = Build Array (concatenate)(w835, w834) -> (w833:i16[])
                    n405 = Build Array (concatenate)(w832, w831) -> (w830:path[])
                  }
                  frame True {
                  }
                }
              }
              frame "Raw voltage" {
              }
            }
          }
          n406 = call "Current_Calib_Filenames.vi"("Calib Filename"=w806, "Channel Numbers"=w807, "Mode"=App_Global."Write to Global") -> ()  [unwired: 3 out]
        }
        frame "Post Process Raw Data File" {
          n407 = for {
            tunnel: w846 -> [w852] mode=indexing
            tunnel: [w851] -> w840 mode=indexing
            n408 = Unbundle By Name(w852) -> ("Calib filename"=w851:path)
          }
          n409 = global read "Meas_global.vi" "Pre Setup String"() -> (w845:string)
          n410 = call "Get_Characters_from_string.vi"("Input string"=w845, "Variable name"="Skip_Block_Numbers_(eg 1;2;5;12)") -> ("Status"=w843:enum16{"Char in string", "Char not in string"}, "Value"=w842:string)  [unwired: 1 in]
          n411 = case shown="\"Char in string\"" w843 {
            tunnel: w842 -> [w849 _]
            tunnel: [w847 i32[] []] -> w841
            frame "Char in string" {
              n412 = call "Get_array_values_fr_String.vi"("String Value"=w849) -> ("Numeric Array"=w848:dbl[])  [unwired: 1 out]
              n413 = To Long Integer(number=w848) -> (32bit integer=w847:i32[])
            }
            frame "Char not in string" {
            }
          }
          n414 = global write "Meas_global.vi" "Blocks to Skip"(w841) -> ()
        }
      }
    }
    frame #8 {
      n415 = global read "Meas_global.vi" "Pre Setup String"() -> (w853:string)
      n416 = for {
        tunnel: [w864] -> w856 mode=indexing
        tunnel: w855 -> [w861] mode=indexing
        tunnel: w854 -> [w863] mode=indexing
        tunnel: w853 -> [w862]
        n417 = Unbundle By Name(w861) -> ("Code name"=w860:string)
        n418 = Concatenate Strings(w860, "_Av_SamplingRate" ("string")) -> (w858:string)
        n419 = call "Get_value_from_string.vi"("Input string"=w862, "Variable name"=w858) -> ("Value"=w857:dbl)  [unwired: 1 in, 1 out]
        n420 = Bundle By Name(cluster=w861, "Calib File"=w863, "Av Sampling Rate"=w857) -> (w864:T8)
      }
      "Analysis Info cluster" <- w856
    }
  }
